vi "取像框架.vi"() -> ()   [LabVIEW 2015]
uses:
  <vilib>/userdefined/High Color/IMAQdx.ctl
  <vilib>/vision/driver/NI_Vision_Acquisition_Software.lvlib
  <vilib>/vision/NI_Vision_Development_Module.lvlib
panel:
  in  "SearchArea":dbl(slide)=0.5 scale=0.0..0.5
  in  "Axis":bool
  out "error out 2":errorcluster
  out "ROI":T1
  in  "開圖":bool=TRUE
  in  "影像數量":i32=1
  in  "Slide":i16(slide) min=0
  in  "Session In":T2="cam1"
  in  "重新開圖":bool
  in  "取像":bool
  out "error out":errorcluster
  in  "stop":bool
  out "Image":T3(plugin-control)
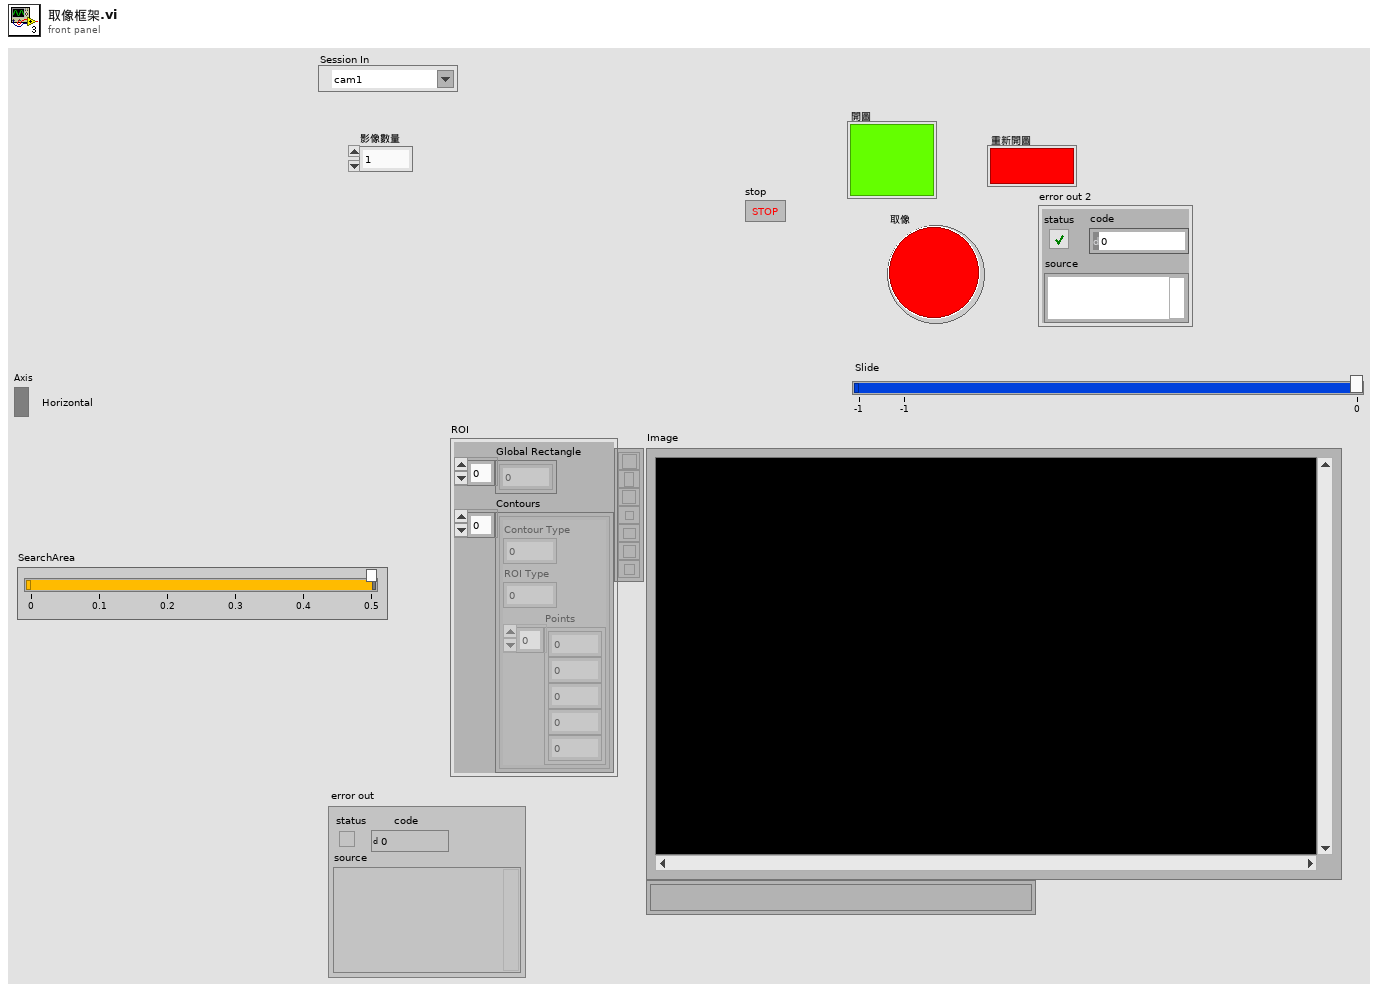
[diagram p1: front panel]
types:
  T1 = cluster{"Global Rectangle":i32[], "Contours":cluster{"Contour Type":u32, "ROI Type":u32, "Points":i32[]}[]}
  T2 = typedef "IMAQdx.ctl" = refnum<k21>
  T3 = typedef "IMAQ Image.ctl" = refnum<image>
  T4 = typedef "IMAQ Rectangle" = cluster{"Left":i32, "Top":i32, "Right":i32, "Bottom":i32, "Rotation":dbl}
  T5 = typedef "ROI Descriptor" = cluster{"Global Rectangle":i32[], "Contours":cluster{"ID":enum32{"External", "Internal"}, "Type":u32, "Coordinates":i32[]}[]}
  T6 = cluster{"Global Rectangle":i32[], "Contours":cluster{"ID":enum32{"External", "Internal"}, "Type":u32, "Coordinates":i32[]}[]}
  T7 = cluster{"Left":i32, "Top":i32, "Right":i32, "Bottom":i32}
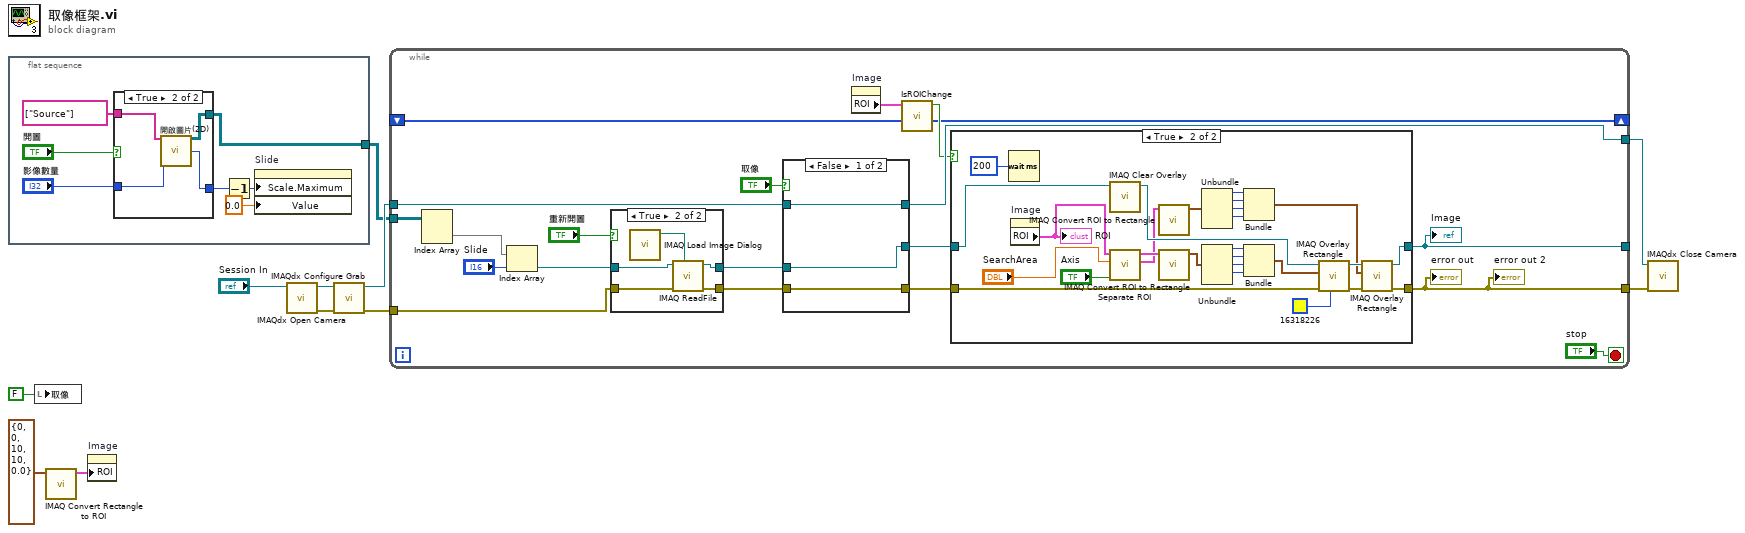
[diagram p0: block diagram]
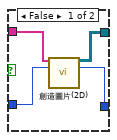
[diagram p2: hidden frame]
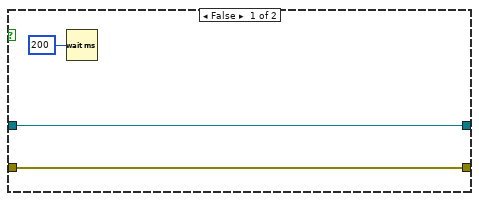
[diagram p4: hidden frame]
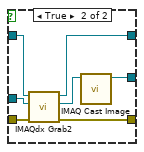
[diagram p5: hidden frame]
diagram:
  n1 = flat-sequence {
    tunnel: [w12] -> w1
    frame #0 {
      n2 = case shown="True" "開圖" {
        tunnel: string[] ["Source"] -> [w20 w26]
        tunnel: [w21 w25] -> w12
        tunnel: [w22 w24] -> w16
        tunnel: "影像數量" -> [w19 w23]
        frame False {
          n3 = call "創造圖片(2D).vi"("ImageNameArray"=w20, "影像數量"=w19) -> ("Image2DArray"=w21:T3[][], "ImageNameNumber"=w22:i32)  [unwired: 10 in, 2 out]
        }
        frame True {
          n4 = call "開啟圖片(2D).vi"("ImageNameArray"=w26, "影像數量"=w23) -> ("Image2DArray"=w25:T3[][], "ImagePathNumber"=w24:i32)  [unwired: 9 in, 3 out]
        }
      }
      n5 = Decrement(x=w16) -> (x-1=w17:i32)
      n6 = property on="Slide" class="Slide (strict)"("Scale.Maximum"=w17, "Value"=0.0 ("Scale.Range:Minimum")) -> ()  [unwired: 2 in, 2 out]
    }
  }
  n7 = local write "取像"(FALSE ("取像")) -> ()
  n8 = call "IMAQ Convert Rectangle to ROI"("Rectangle"=T4 {"Left"=0, "Top"=0, "Right"=10, "Bottom"=10, "Rotation"=0.0}) -> ("ROI Descriptor"=w5:T5)  [unwired: 8 in, 1 out]
  n9 = property on="Image" class="ImageControl"("ROI"=w5) -> ()  [unwired: 2 in, 2 out]
  n10 = call <vilib>:"IMAQdx Open Camera.vi"("Session In"="Session In") -> ("error out"=w7:errorcluster, "Session Out"=w8:T2)  [unwired: 9 in]
  n11 = call <vilib>:"IMAQdx Configure Grab.vi"("error in"=w7, "Session In"=w8) -> ("error out"=w3:errorcluster, "Session Out"=w11:T2)  [unwired: 8 in]
  n12 = while {
    tunnel: w11 -> [w46]
    tunnel: w1 -> [w34]
    tunnel: [w44] -> w10
    tunnel: [w27] -> _
    tunnel: w3 -> [w40]
    tunnel: [w39] -> w2
    shift-right: [w29] -> _
    shift-left: _ -> [w28]
    stop <- "stop" stop-if-true
    n13 = Index Array(array=w34) -> (element=w35:T3[])  [unwired: 2 in]
    n14 = Index Array(array=w35, index="Slide") -> (element=w33:T3)
    n15 = case shown="True" "重新開圖" {
      tunnel: w33 -> [w48 w51]
      tunnel: [w48 w52] -> w42
      tunnel: w40 -> [w47 w50]
      tunnel: [w47 w49] -> w38
      frame False {
      }
      frame True {
        n16 = call "IMAQ Load Image Dialog"() -> ("Path"=w53:path)  [unwired: 9 in, 2 out]
        n17 = call "IMAQ ReadFile"("File Path"=w53, "error in (no error)"=w50, "Image"=w51) -> ("error out"=w49:errorcluster, "Image Out"=w52:T3)  [unwired: 4 in, 3 out]
      }
    }
    n18 = case shown="False" "取像" {
      tunnel: w46 -> [w85 w92]
      tunnel: w42 -> [w84 w91]
      tunnel: [w85 w90] -> w44
      tunnel: [w84 w87] -> w36
      tunnel: w38 -> [w83 w89]
      tunnel: [w83 w88] -> w41
      frame False {
      }
      frame True {
        n19 = call <vilib>:"IMAQdx Grab2.vi"("error in"=w89, "Image In"=w91, "Session In"=w92) -> ("error out"=w88:errorcluster, "Image Out"=w86:T3, "Session Out"=w90:T2)  [unwired: 5 in, 1 out]
        n20 = call "IMAQ Cast Image"("Image Src"=w86) -> ("Image Dst Out"=w87:T3)  [unwired: 9 in, 1 out]
      }
    }
    n21 = property on="Image" class="ImageControl"() -> ("ROI"=w31:T1)  [unwired: 2 in, 2 out]
    n22 = call "IsROIChange.vi"("InputData"=w28, "ROI"=w31) -> ("OutputData"=w29:u32[], "Change?"=w30:bool)  [unwired: 8 in]
    n23 = case shown="True" w30 {
      tunnel: w41 -> [w56 w64]
      tunnel: w36 -> [w55 w81]
      tunnel: [w55 w68] -> w27
      tunnel: [w56 w63] -> w39
      frame False {
        n24 = Wait (ms)(milliseconds to wait=u32 200) -> ()  [unwired: 1 out]
      }
      frame True {
        n25 = Wait (ms)(milliseconds to wait=u32 200) -> ()  [unwired: 1 out]
        n26 = property on="Image" class="ImageControl"() -> ("ROI"=w62:T1)  [unwired: 2 in, 2 out]
        "ROI" <- w62
        n27 = call "IMAQ Clear Overlay"("Image"=w81) -> ("Image Out"=w69:T3)  [unwired: 9 in, 1 out]
        n28 = call "Separate ROI.vi"("Axis"="Axis", "SearchArea"="SearchArea", "ROI Descriptor"=w62) -> ("Right/Bottom ROI"=w57:T6, "Left/Top ROI"=w58:T6)  [unwired: 3 in]
        n29 = call "IMAQ Convert ROI to Rectangle"("ROI Descriptor"=w57) -> ("Rectangle"=w79:T4)  [unwired: 8 in, 1 out]
        n30 = call "IMAQ Convert ROI to Rectangle"("ROI Descriptor"=w58) -> ("Rectangle"=w80:T4)  [unwired: 8 in, 1 out]
        n31 = Unbundle(w79) -> ("Left"=w74:i32, "Top"=w73:i32, "Right"=w72:i32, "Bottom"=w71:i32)  [unwired: 1 out]
        n32 = Unbundle(w80) -> ("Left"=w78:i32, "Top"=w77:i32, "Right"=w76:i32, "Bottom"=w75:i32)  [unwired: 1 out]
        n33 = Bundle("Left"=w74, "Top"=w73, "Right"=w72, "Bottom"=w71) -> (w66:T7)  [unwired: 1 in]
        n34 = Bundle("Left"=w78, "Top"=w77, "Right"=w76, "Bottom"=w75) -> (w67:T7)  [unwired: 1 in]
        n35 = call "IMAQ Overlay Rectangle"("Color"=u32 16318226, "error in (no error)"=w64, "Rectangle"=w67, "Image"=w69) -> ("error out"=w65:errorcluster, "Image Out"=w70:T3)  [unwired: 6 in]
        n36 = call "IMAQ Overlay Rectangle"("error in (no error)"=w65, "Rectangle"=w66, "Image"=w70) -> ("error out"=w63:errorcluster, "Image Out"=w68:T3)  [unwired: 7 in]
      }
    }
    "Image" <- w27
    "error out" <- w39
    "error out 2" <- w39
  }
  n37 = call <vilib>:"IMAQdx Close Camera.vi"("error in"=w2, "Session In"=w10) -> ()  [unwired: 9 in, 1 out]
